vi "Draw PDO Mappings.vi"(7 "PDO Mappables":string[](array[string]), 8 "error in":errorcluster, 9 "PDO Slot in":refnum<class "PDO Slot.lvclass">, 10 "Row":i32, 11 "PDO Grid in":refnum<class "PDO Grid.lvclass">) -> (0 "error out":errorcluster, 3 "PDO Grid out":refnum<class "PDO Grid.lvclass">)   [LabVIEW 2020, in "PDO Grid.lvlib" / "PDO Grid.lvclass"]
uses:
  PDO Grid.lvclass
  D:/git/Sourcegrid-LabVIEW/source/Grid/SourceGrid.lvclass
  PDO Slot/PDO Slot.lvclass
  Sourcegrid-LabVIEW/source/Cells/Cell/Cell.lvclass
  Sourcegrid-LabVIEW/source/Editors/Combo Box/Combo Box.lvclass
  D:/git/Sourcegrid-LabVIEW/source/Editors/Editor Base/Editor Control Base.lvclass
  PDO Slot/PDO Slot.lvclass/PDO Slot.ctl
  PDO Mapping/PDO Mapping.lvclass/PDO Mapping.ctl
  Sourcegrid-LabVIEW/source/Views/Cell View Alternating Back Color/Cell View Alternating Back Color.lvclass
  D:/git/Sourcegrid-LabVIEW/source/Views/Cell View/Cell View.lvclass
  PDO Mapping/PDO Mapping.lvclass
  Core/OD Entry/OD Entry.lvclass
  Sourcegrid-LabVIEW/source/System.Drawing.Color.ctl
  Sourcegrid-LabVIEW/source/SourceGrid.lvlib
  Sourcegrid-LabVIEW/source/Grid/SourceGrid.lvclass
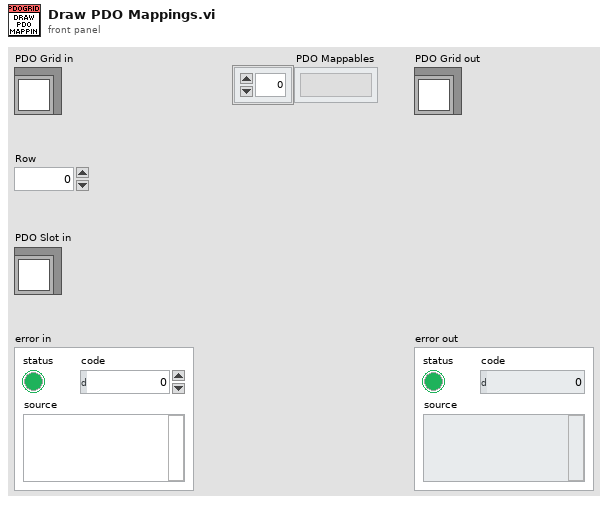
[diagram p1: front panel]
types:
  T1 = typedef "SourceGrid.lvlib/System.Drawing.Color.ctl" = enum16{"AliceBlue", "AntiqueWhite", "Aqua", "Aquamarine", "Azure", "Beige", "Bisque", "Black", "BlanchedAlmond", "Blue", "BlueViolet", "Brown", "BurlyWood", "CadetBlue", "Chartreuse", "Chocolate", "Coral", "CornflowerBlue", "Cornsilk", "Crimson", "Cyan", "DarkBlue", "DarkCyan", "DarkGoldenrod", "DarkGray", "DarkGreen", "DarkKhaki", "DarkMagenta", "DarkOliveGreen", "DarkOrange", "DarkOrchid", "DarkRed", "DarkSalmon", "DarkSeaGreen", "DarkSlateBlue", "DarkSlateGray", "DarkTurquoise", "DarkViolet", "DeepPink", "DeepSkyBlue", "DimGray", "DodgerBlue", "Firebrick", "FloralWhite", "ForestGreen", "Fuchsia", "Gainsboro", "GhostWhite", "Gold", "Goldenrod", "Gray", "Green", "GreenYellow", "Honeydew", "HotPink", "IndianRed", "Indigo", "Ivory", "Khaki", "Lavender", "LavenderBlush", "LawnGreen", "LemonChiffon", "LightBlue", "LightCoral", "LightCyan", "LightGoldenrodYellow", "LightGray", "LightGreen", "LightPink", "LightSalmon", "LightSeaGreen", "LightSkyBlue", "LightSlateGray", "LightSteelBlue", "LightYellow", "Lime", "LimeGreen", "Linen", "Magenta", "Maroon", "MediumAquamarine", "MediumBlue", "MediumOrchid", "MediumPurple", "MediumSeaGreen", "MediumSlateBlue", "MediumSpringGreen", "MediumTurquoise", "MediumVioletRed", "MidnightBlue", "MintCream", "MistyRose", "Moccasin", "NavajoWhite", "Navy", "OldLace", "Olive", "OliveDrab", "Orange", "OrangeRed", "Orchid", "PaleGoldenrod", "PaleGreen", "PaleTurquoise", "PaleVioletRed", "PapayaWhip", "PeachPuff", "Peru", "Pink", "Plum", "PowderBlue", "Purple", "Red", "RosyBrown", "RoyalBlue", "SaddleBrown", "Salmon", "SandyBrown", "SeaGreen", "SeaShell", "Sienna", "Silver", "SkyBlue", "SlateBlue", "SlateGray", "Snow", "SpringGreen", "SteelBlue", "Tan", "Teal", "Thistle", "Tomato", "Transparent", "Turquoise", "Violet", "Wheat", "White", "WhiteSmoke", "Yellow"}
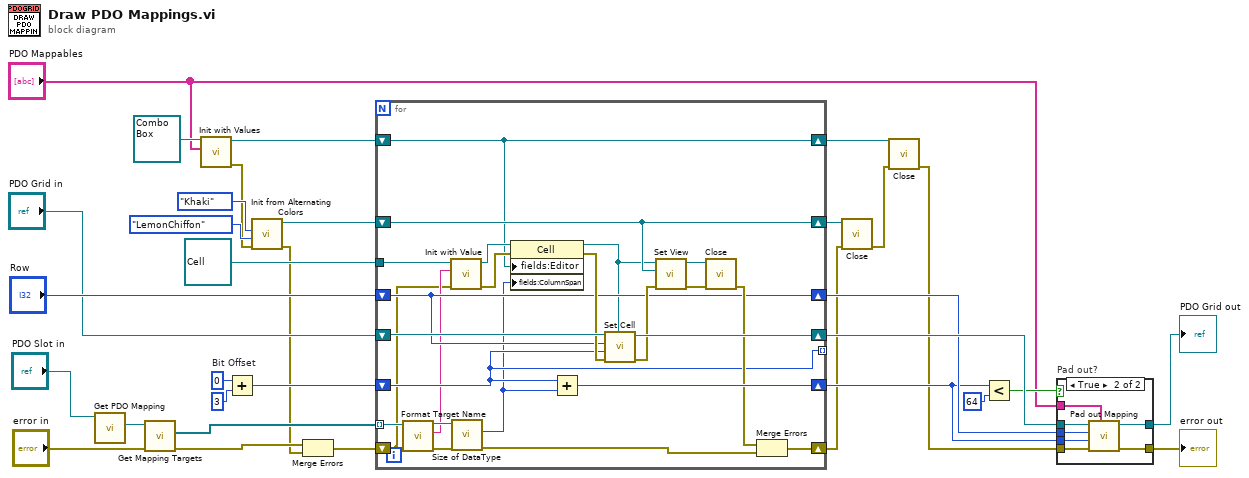
[diagram p0: block diagram]
diagram:
  w29 = 0  # Bit Offset
  n1 = call "Get PDO Mapping.vi"("PDO Slot in"="PDO Slot in") -> ("PDO Grid.lvlib:PDO Mapping"=w23:refnum<class "PDO Mapping.lvclass">)  [unwired: 8 in, 2 out]
  n2 = call "Get Mapping Targets.vi"("error in (no error)"="error in", "PDO Mapping in"=w23) -> ("error out"=w28:errorcluster, "Mapping Targets"=w27:refnum<class "OD Entry.lvclass">[])  [unwired: 7 in, 1 out]
  n3 = call-dynamic "Init with Values.vi"("Values"="PDO Mappables", "Combo Box in"=refnum<class "Combo Box.lvclass"> refnum ("SourceGrid.lvlib:Combo Box.lvclass")) -> ("error out"=w3:errorcluster, "Combo Box out"=w6:refnum<class "Combo Box.lvclass">)  [unwired: 8 in]
  n4 = Add(x=w29, y=3) -> (x+y=w30:i32)
  n5 = call "Init from Alternating Colors.vi"("error in"=w3, "Color Not Equal"=System.Drawing.Color."LemonChiffon" ("Color"), "Color Equal"=System.Drawing.Color."Khaki" ("Color")) -> ("error out"=w8:errorcluster, "Cell View Alternating Back Color out"=w21:refnum<class "Cell View Alternating Back Color.lvclass">)  [unwired: 7 in]
  n6 = Merge Errors(w28, w8) -> (w9:errorcluster)
  n7 = for {
    tunnel: w27 -> [w52] mode=indexing
    shift-right: [w48] -> w10
    shift-left: w9 -> [w34]
    shift-right: [w49] -> w14
    shift-left: w30 -> [w43]
    tunnel: refnum<class "Cell.lvclass"> refnum ("SourceGrid.lvlib:Cell.lvclass") -> [w55]
    shift-right: [w50] -> w26
    shift-left: "PDO Grid in" -> [w56]
    tunnel: [w43] -> _ mode=indexing
    shift-right: [w44] -> w16
    shift-left: "Row" -> [w44]
    shift-right: [w39] -> w18
    shift-left: w21 -> [w39]
    shift-right: [w35] -> w4
    shift-left: w6 -> [w35]
    n8 = call "Format Target Name.vi"("error in"=w34, "OD Entry in"=w52) -> ("error out"=w53:errorcluster, "Name"=w42:string, "OD Entry out"=w51:refnum<class "OD Entry.lvclass">)  [unwired: 7 in]
    n9 = call-dynamic "Init with Value.vi"("error in"=w34, "Value"=w42, "Cell in"=w55) -> ("error out"=w37:errorcluster, "Cell out"=w38:refnum<class "Cell.lvclass">)  [unwired: 7 in]
    n10 = call "Size of DataType.vi"("error in"=w53, "OD Entry in"=w51) -> ("error out"=w47:errorcluster, "Size in Bits"=w36:i32)  [unwired: 7 in, 1 out]
    n11 = property class="Cell"(reference=w38, error in=w37, "fields:Editor"=w35, "fields:ColumnSpan"=w36) -> (reference out=w33:refnum<class "Cell.lvclass">, error out=w54:errorcluster)
    n12 = Add(x=w43, y=w36) -> (x+y=w49:i32)
    n13 = call "Set Cell.vi"("Cell"=w33, "error in"=w54, "Column"=w43, "Row"=w44, "Sourcegrid in"=w56) -> ("error out"=w46:errorcluster, "Sourcegrid out"=w50:refnum<class "PDO Grid.lvclass">)  [unwired: 5 in]
    n14 = call-dynamic "Set View.vi"("error in"=w46, "CellView"=w39, "Cell in"=w33) -> ("error out"=w41:errorcluster, "Cell out"=w40:refnum<class "Cell.lvclass">)  [unwired: 7 in]
    n15 = call-dynamic "Close.vi"("error in"=w41, "Cell in"=w40) -> ("error out"=w45:errorcluster)  [unwired: 8 in, 1 out]
    n16 = Merge Errors(w45, w47) -> (w48:errorcluster)
  }
  n17 = call-dynamic "Close.vi"("error in"=w10, "Cell View Alternating Back Color in"=w18) -> ("error out"=w5:errorcluster)  [unwired: 8 in, 1 out]
  n18 = call-dynamic "Close.vi"("error in"=w5, "Combo Box in"=w4) -> ("error out"=w7:errorcluster)  [unwired: 8 in, 1 out]
  n19 = Less?(x=w14, y=64) -> (x < y?=w12:bool)
  n20 = case "Pad out?" shown="True" w12 {
    tunnel: w26 -> [w57 w65]
    tunnel: [w57 w64] -> w17
    tunnel: w16 -> [_ w63]
    tunnel: w7 -> [w58 w62]
    tunnel: [w58 w61] -> w15
    tunnel: w14 -> [_ w60]
    tunnel: "PDO Mappables" -> [_ w59]
    frame False {
    }
    frame True {
      n21 = call "Pad out Mapping.vi"("PDO Mappables"=w59, "error in"=w62, "Bit Offset"=w60, "Row"=w63, "PDO Grid in"=w65) -> ("error out"=w61:errorcluster, "PDO Grid out"=w64:refnum<class "PDO Grid.lvclass">)  [unwired: 5 in]
    }
  }
  "PDO Grid out" <- w17
  "error out" <- w15
